vi "Get Today Time.vi"(11 "System Time (s)":dbl) -> (3 "Today Time":dbl)   [LabVIEW 2020]
doc: "This VI get today time."
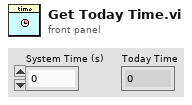
[diagram p1: front panel]
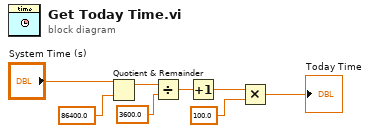
[diagram p0: block diagram]
diagram:
  n1 = Quotient & Remainder(x="System Time (s)", y=86400.0) -> (x-y*floor(x/y)=w2:dbl)  [unwired: 1 out]
  n2 = Divide(x=w2, y=3600.0) -> (x/y=w4:dbl)
  n3 = Increment(x=w4) -> (x+1=w5:dbl)
  n4 = Multiply(x=w5, y=100.0) -> (x*y=→"Today Time":dbl)
